vi "Diag_EntityInfo.vi"(0 "GEA2 Reference In":refnum<k24>, 5 "GEA Inputs":T2={"Source"=228, "Destination"=0} {"Destination" format="%.0x"; "Source" format="%.0x"}, 11 "Error In":errorcluster, 13 "Entity Location":u16 format="%.0x") -> (4 "GEA2 Reference Out":refnum<k24>, 6 "Diagnostic Entity Manifest":T1, 15 "Error Out":errorcluster)   [LabVIEW 2023]
uses:
  D:/Common/LabVIEW GEA2 Toolkit/source/GEA3 DLL Source/GeaCommunication.dll
  LabVIEW GEA2 Toolkit/source/GEA3 DLL Source/GeaCommunication.dll
  LabVIEW GEA2 Toolkit/GEA3/type defs/Source_Destination.ctl
  Type Defs/Diag_EntityManifestType.ctl
  LabVIEW GEA2 Toolkit/GEA3/type defs/ERD Read Data In.ctl
  LabVIEW GEA2 Toolkit/GEA3/library/GEA2_Toolkit.lvlib
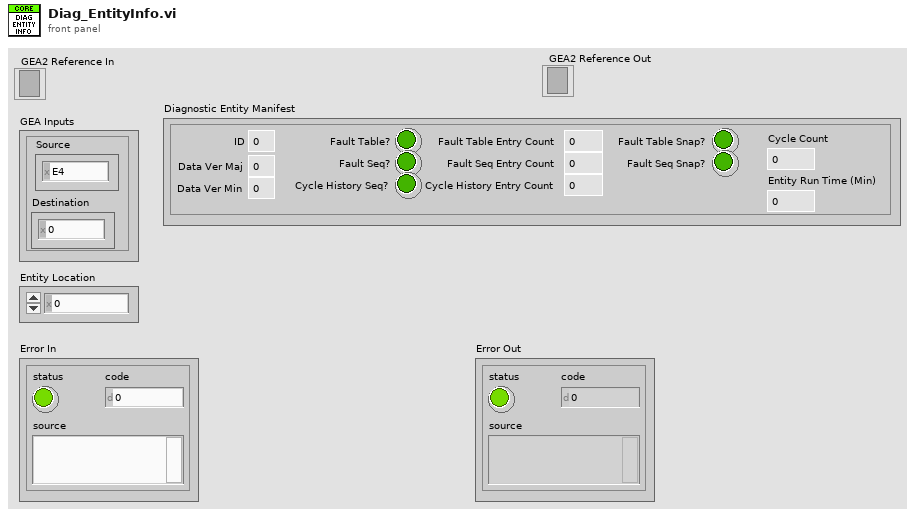
[diagram p1: front panel]
types:
  T1 = typedef "Diag_EntityManifestType.ctl" = cluster{"ID":u8, "Data Ver Maj":u8, "Data Ver Min":u8, "Fault Table?":bool, "Fault Table Snap?":bool, "Fault Seq?":bool, "Fault Seq Snap?":bool, "Cycle History Seq?":bool, "Fault Table Entry Count":u16, "Fault Seq Entry Count":u16, "Cycle History Entry Count":u16, "Cycle Count":u32, "Entity Run Time (Min)":u32}
  T2 = typedef "Source_Destination.ctl" = cluster{"Source":u8, "Destination":u8}
  T3 = typedef "ERD Read Data In.ctl" = cluster{"ERD Number":u16, "Data Type":enum16{"string", "boolean", "uint8_t", "uint16_t", "uint32_t", "uint64_t", "int8_t", "int16_t", "int32_t", "int64_t"}}
  T4 = typedef "ERD Read Data Out.ctl" = cluster{"ERD Number":u16, "Data":string}
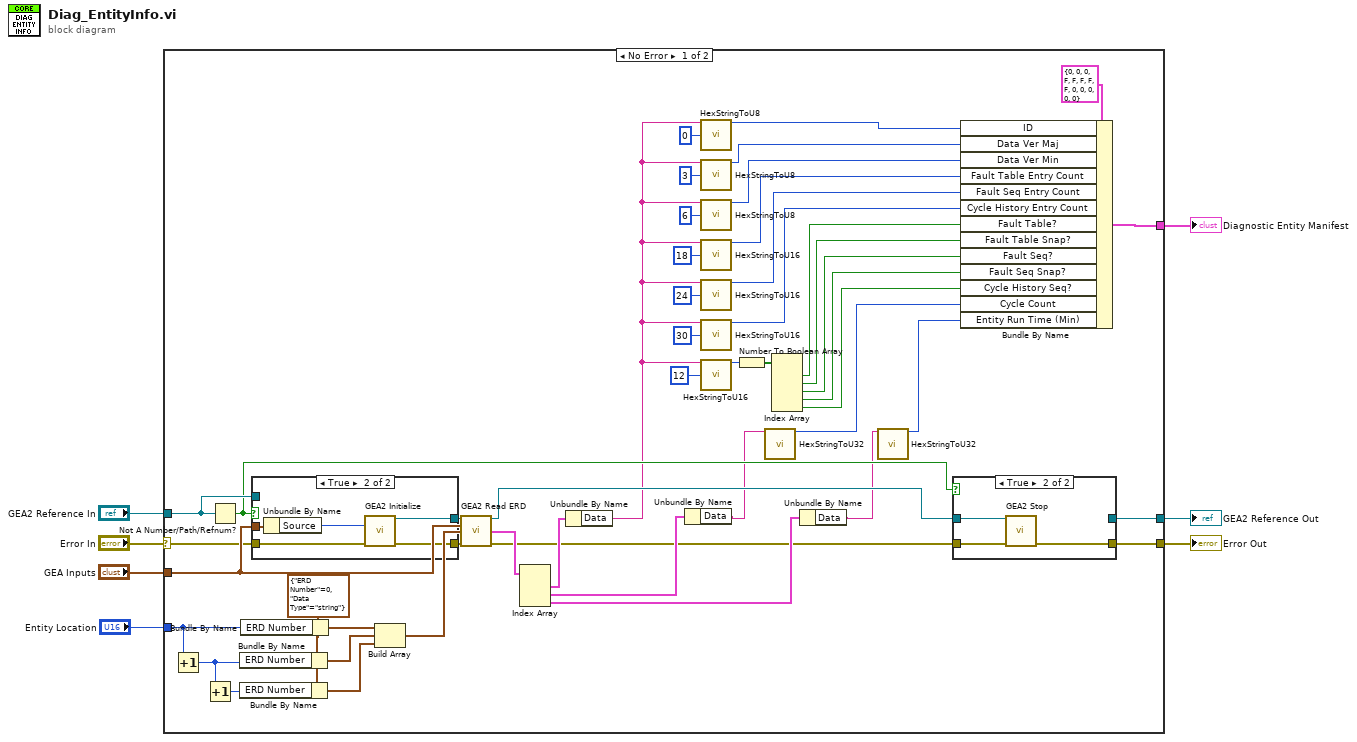
[diagram p0: block diagram]
diagram:
  n1 = case shown="No Error" "Error In" {
    selector: "Error In" -> [w47 w70]
    tunnel: [w46 w70] -> w7
    tunnel: "GEA2 Reference In" -> [w56 w69]
    tunnel: "GEA Inputs" -> [w51 _]
    tunnel: [w48 w69] -> w4
    tunnel: "Entity Location" -> [w43 _]
    tunnel: [w35 _] -> w1
    frame No Error {
      w45 = T3 {"ERD Number"=0, "Data Type"=enum."string"} ("ERD Read Data In")
      n2 = Increment(x=w43) -> (x+1=w8:u16)
      n3 = Increment(x=w8) -> (x+1=w44:u16)
      n4 = Not A Number/Path/Refnum?(number/path/refnum=w56) -> (NaN/Path/Refnum?=w49:bool)
      n5 = Bundle By Name(cluster=w45, "ERD Number"=w8) -> (w41:T3)
      n6 = Bundle By Name(cluster=w45, "ERD Number"=w44) -> (w40:T3)
      n7 = Bundle By Name(cluster=w45, "ERD Number"=w43) -> (w42:T3)
      n8 = case shown="True" w49 {
        tunnel: w47 -> [w62 w68]
        tunnel: w51 -> [_ w67]
        tunnel: [w62 w66] -> w55
        tunnel: [w63 w65] -> w54
        tunnel: w56 -> [w63 _]
        frame False {
        }
        frame True {
          n9 = Unbundle By Name(w67) -> ("Source"=w64:u8)
          n10 = call "GEA2 Initialize.vi"("Source Address"=w64, "error in"=w68) -> ("GEA2 Reference Out"=w65:refnum<k24>, "error out"=w66:errorcluster)  [unwired: 10 in, 2 out]
        }
      }
      n11 = Build Array(w42, w41, w40) -> (w39:T3[])
      n12 = call "GEA2 Read ERD.vi"("GEA2 Reference In"=w54, "GEA Inputs"=w51, "Read ERD List"=w39, "Error In"=w55) -> ("GEA2 Reference Out"=w50:refnum<k24>, "ERD Data Out"=w53:T4[], "Error Out"=w9:errorcluster)  [unwired: 8 in, 1 out]
      n13 = Index Array(array=w53) -> (element #1=w52:T4, element #2=w38:T4, element #3=w37:T4)  [unwired: 3 in]
      n14 = Unbundle By Name(w52) -> ("Data"=w12:string)
      n15 = Unbundle By Name(w38) -> ("Data"=w11:string)
      n16 = call "HexStringToU8.vi"("Input String"=w12, "Starting Offset"=0) -> ("Number Out"=w26:u8)  [unwired: 13 in]
      n17 = call "HexStringToU8.vi"("Input String"=w12, "Starting Offset"=3) -> ("Number Out"=w25:u8)  [unwired: 13 in]
      n18 = call "HexStringToU8.vi"("Input String"=w12, "Starting Offset"=6) -> ("Number Out"=w24:u8)  [unwired: 13 in]
      n19 = call "HexStringToU16.vi"("Input String"=w12, "Starting Offset"=18) -> ("Number Out"=w23:u16)  [unwired: 13 in]
      n20 = call "HexStringToU16.vi"("Input String"=w12, "Starting Offset"=24) -> ("Number Out"=w22:u16)  [unwired: 13 in]
      n21 = call "HexStringToU16.vi"("Input String"=w12, "Starting Offset"=30) -> ("Number Out"=w21:u16)  [unwired: 13 in]
      n22 = call "HexStringToU16.vi"("Input String"=w12, "Starting Offset"=12) -> ("Number Out"=w20:u16)  [unwired: 13 in]
      n23 = Number To Boolean Array(number=w20) -> (Boolean array=w19:bool[])
      n24 = call "HexStringToU32.vi"("Input String"=w11) -> ("Number Out"=w27:u32)  [unwired: 14 in]
      n25 = Index Array(array=w19) -> (element #1=w17:bool, element #2=w16:bool, element #3=w15:bool, element #4=w14:bool, element #5=w13:bool)  [unwired: 5 in]
      n26 = Unbundle By Name(w37) -> ("Data"=w10:string)
      n27 = call "HexStringToU32.vi"("Input String"=w10) -> ("Number Out"=w28:u32)  [unwired: 14 in]
      n28 = case shown="True" w49 {
        tunnel: w9 -> [w57 w61]
        tunnel: [w57 w60] -> w46
        tunnel: [w58 _] -> w48
        tunnel: w50 -> [w58 w59]
        frame False {
        }
        frame True {
          n29 = call "GEA2 Stop.vi"("GEA2 Reference In"=w59, "Error In"=w61) -> ("Error Out"=w60:errorcluster)  [unwired: 13 in]
        }
      }
      n30 = Bundle By Name(cluster=T1 {"ID"=0, "Data Ver Maj"=0, "Data Ver Min"=0, "Fault Table?"=FALSE, "Fault Table Snap?"=FALSE, "Fault Seq?"=FALSE, "Fault Seq Snap?"=FALSE, "Cycle History Seq?"=FALSE, "Fault Table Entry Count"=0, "Fault Seq Entry Count"=0, "Cycle History Entry Count"=0, "Cycle Count"=0, "Entity Run Time (Min)"=0} ("Diagnostic Entity Manifest"), "ID"=w26, "Data Ver Maj"=w25, "Data Ver Min"=w24, "Fault Table Entry Count"=w23, "Fault Seq Entry Count"=w22, "Cycle History Entry Count"=w21, "Fault Table?"=w17, "Fault Table Snap?"=w16, "Fault Seq?"=w15, "Fault Seq Snap?"=w14, "Cycle History Seq?"=w13, "Cycle Count"=w27, "Entity Run Time (Min)"=w28) -> (w35:T1)
    }
    frame Error {
    }
  }
  "Error Out" <- w7
  "GEA2 Reference Out" <- w4
  "Diagnostic Entity Manifest" <- w1
